vi "Config.vi"(8 "error in (no error)":errorcluster, 10 "URL":string, 11 "Firebase in":refnum<class "Firebase.lvclass">) -> (0 "error out":errorcluster, 3 "Firebase out":refnum<class "Firebase.lvclass">)   [LabVIEW 2019, in "Firebase.lvclass"]
uses:
  Firebase.lvclass
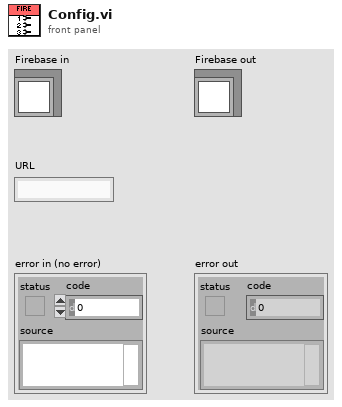
[diagram p1: front panel]
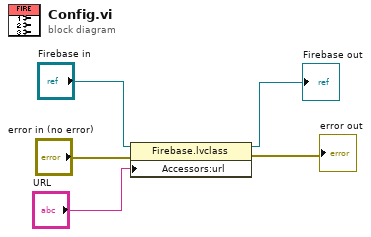
[diagram p0: block diagram]
diagram:
  n1 = property class="Firebase.lvclass"(reference="Firebase in", error in="error in (no error)", "Accessors:url"="URL") -> (reference out=→"Firebase out":refnum<class "Firebase.lvclass">, error out=→"error out":errorcluster)
